vi "E4980ALsettingsAF.vi"(9 "Frequency, Hz":dbl=1000.0, 10 "Amplitude, V":dbl=100.0, 11 "VISA resource name":refnum<visa-resource-name>) -> (1 "OUTFrequency":dbl, 2 "OUTAmplitude":dbl, 3 "VISA resource name out":refnum<visa-resource-name>)   [LabVIEW 2017]
panel:
  # "от 0 до 2000 мВ, через 0.1 мВ\n\nпо умолчанию 100мВ"
  # "от 20 до 300000 Гц\n\nпо умолчанию 1000 Гц"
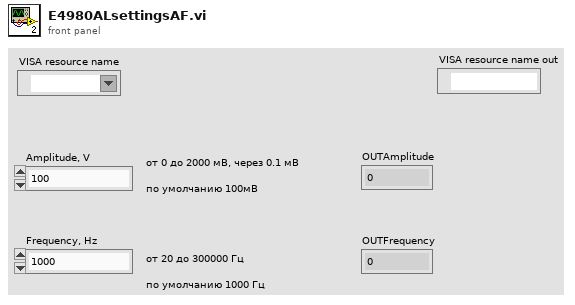
[diagram p1: front panel]
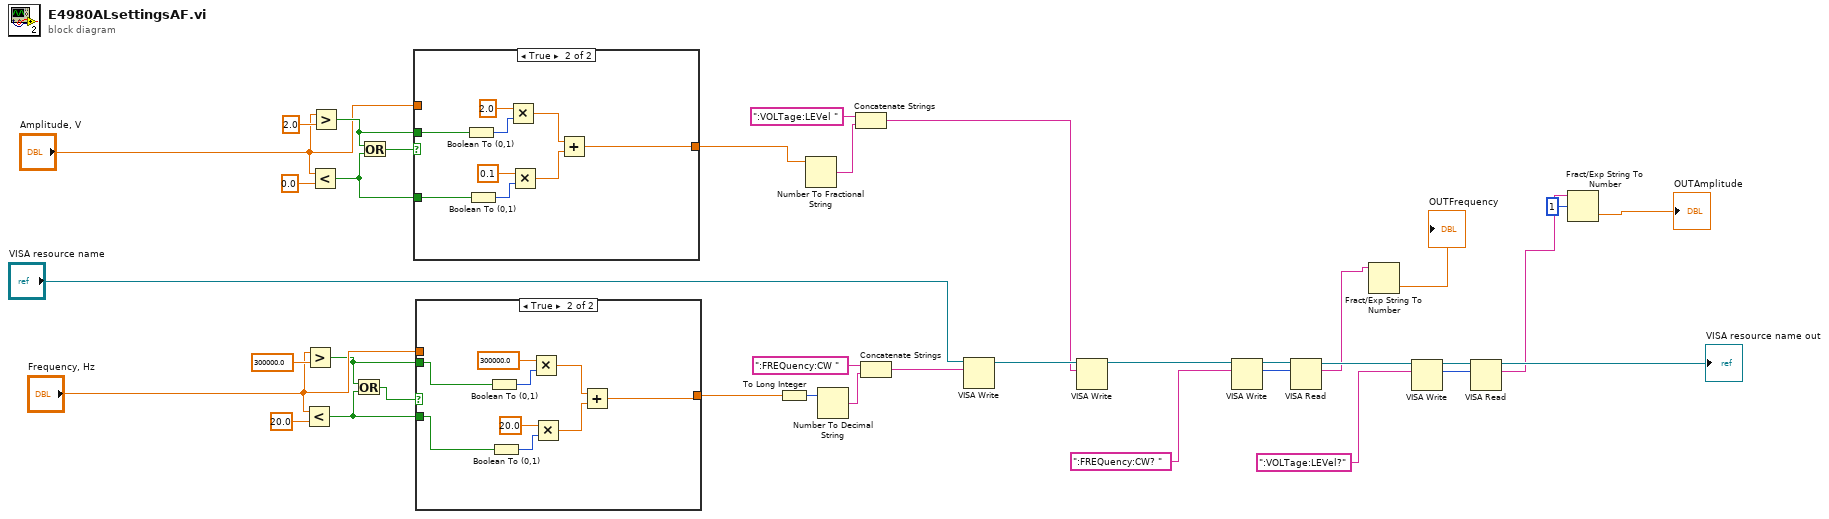
[diagram p0: block diagram]
diagram:
  n1 = Less?(x="Frequency, Hz", y=20.0) -> (x < y?=w27:bool)
  n2 = Greater?(x="Frequency, Hz", y=300000.0) -> (0:w28:bool)
  n3 = Less?(x="Amplitude, V", y=0.0) -> (x < y?=w29:bool)
  n4 = Greater?(x="Amplitude, V", y=2.0) -> (0:w30:bool)
  n5 = Or(x=w28, y=w27) -> (x .or. y?=w32:bool)
  n6 = Or(x=w30, y=w29) -> (x .or. y?=w35:bool)
  n7 = case shown="True" w35 {
    tunnel: "Amplitude, V" -> [w38 _]
    tunnel: w30 -> [_ w40]
    tunnel: w29 -> [_ w39]
    tunnel: [w38 w41] -> w8
    frame False {
    }
    frame True {
      n8 = Boolean To (0,1)(Boolean=w40) -> (0, 1=w44:i16)
      n9 = Boolean To (0,1)(Boolean=w39) -> (0, 1=w45:i16)
      n10 = Multiply(x=2.0, y=w44) -> (x*y=w46:dbl)
      n11 = Multiply(x=0.1, y=w45) -> (x*y=w47:dbl)
      n12 = Add(x=w46, y=w47) -> (x+y=w41:dbl)
    }
  }
  n13 = case shown="True" w32 {
    tunnel: "Frequency, Hz" -> [w48 _]
    tunnel: w28 -> [_ w50]
    tunnel: w27 -> [_ w49]
    tunnel: [w48 w51] -> w23
    frame False {
    }
    frame True {
      n14 = Boolean To (0,1)(Boolean=w50) -> (0, 1=w57:i16)
      n15 = Boolean To (0,1)(Boolean=w49) -> (0, 1=w56:i16)
      n16 = Multiply(x=300000.0, y=w57) -> (x*y=w55:dbl)
      n17 = Multiply(x=20.0, y=w56) -> (x*y=w54:dbl)
      n18 = Add(x=w55, y=w54) -> (x+y=w51:dbl)
    }
  }
  n19 = To Long Integer(number=w23) -> (32bit integer=w25:i32)
  n20 = Number To Fractional String(number=w8) -> (F-format string=w9:string)  [unwired: 3 in]
  n21 = Number To Decimal String(number=w25) -> (decimal integer string=w24:string)  [unwired: 1 in]
  n22 = Concatenate Strings(":VOLTage:LEVel " ("string"), w9) -> (w18:string)
  n23 = Concatenate Strings(":FREQuency:CW " ("string"), w24) -> (w22:string)
  n24 = VISA Write(VISA resource name="VISA resource name", write buffer=w22) -> (VISA resource name out=w20:refnum<visa-resource-name>)  [unwired: 1 in, 2 out]
  n25 = VISA Write(VISA resource name=w20, write buffer=w18) -> (VISA resource name out=w17:refnum<visa-resource-name>)  [unwired: 1 in, 2 out]
  n26 = VISA Write(VISA resource name=w17, write buffer=":FREQuency:CW? " ("string")) -> (VISA resource name out=w15:refnum<visa-resource-name>, return count=w14:u32)  [unwired: 1 in, 1 out]
  n27 = VISA Read(VISA resource name=w15, byte count=w14) -> (VISA resource name out=w11:refnum<visa-resource-name>, read buffer=w6:string)  [unwired: 1 in, 2 out]
  n28 = Fract/Exp String To Number(string=w6) -> (number=→"OUTFrequency":dbl)  [unwired: 3 in, 1 out]
  n29 = VISA Write(VISA resource name=w11, write buffer=":VOLTage:LEVel?" ("string")) -> (VISA resource name out=w10:refnum<visa-resource-name>, return count=w12:u32)  [unwired: 1 in, 1 out]
  n30 = VISA Read(VISA resource name=w10, byte count=w12) -> (VISA resource name out=→"VISA resource name out":refnum<visa-resource-name>, read buffer=w5:string)  [unwired: 1 in, 2 out]
  n31 = Fract/Exp String To Number(string=w5, offset=1) -> (number=→"OUTAmplitude":dbl)  [unwired: 2 in, 1 out]
